vi "dB.vi"(8 "error in (no error)":errorcluster, 11 "Modulo a obtener":T1=enum."Error") -> (0 "error out":errorcluster)   [LabVIEW 2020]
uses:
  Comunes/Controles/Lista Modulos.ctl
  Comunes/Controles/FGV Opciones.ctl
  Comunes/Controles/Sql.ctl
  Comunes/Comunicacion/Mensajes.lvlib
types:
  T1 = typedef "Lista Modulos.ctl" = enum16{"Math", "Error", "Front", "Database", "Nuevos items"}
  T2 = typedef "FGV Opciones.ctl" = enum16{"Get", "Create", "Destroy"}
  T3 = enum32{"Invalid", "Standard", "Closed", "Hidden", "Minimized", "Maximized"}
  T4 = typedef "Sql.ctl" = enum16{"Get zapatos", "Insrt Zapatos", "Insrt Elementos", "Borrar Elementos"}
  T5 = cluster{"Fecha de termino":timestamp, "Fecha de inicio":timestamp, "Modelo":string, "Talla":string, "Color":string}
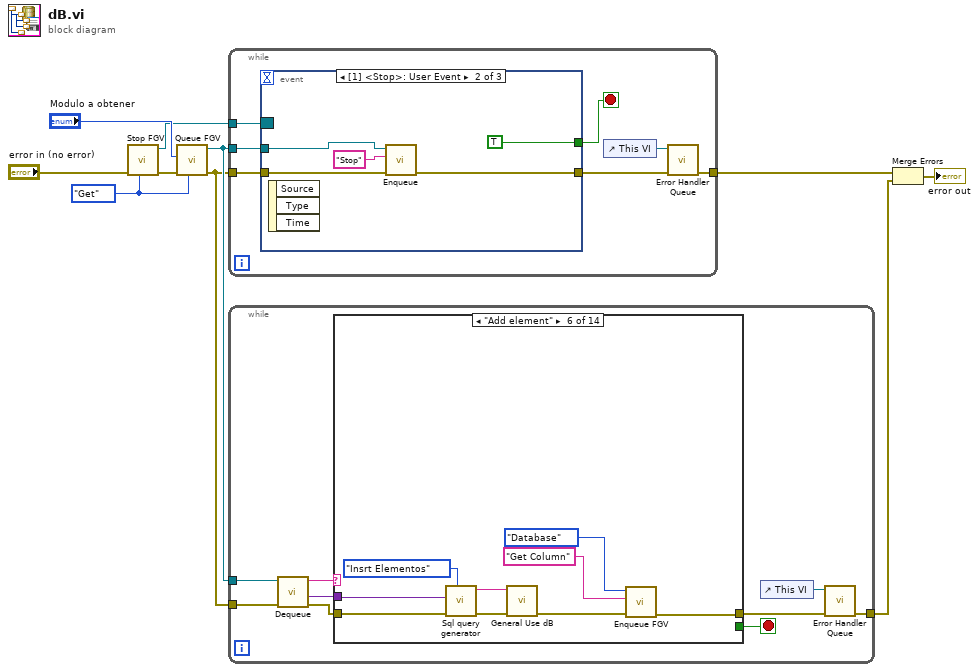
[diagram p0: block diagram]
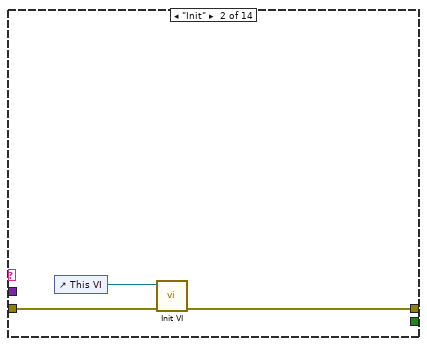
[diagram p3: hidden frame]
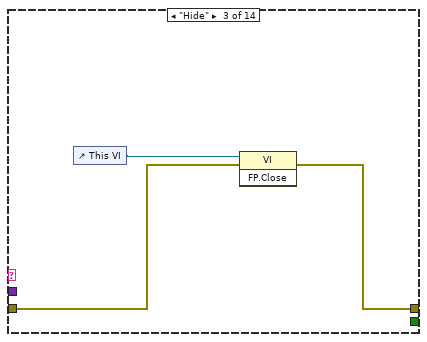
[diagram p4: hidden frame]
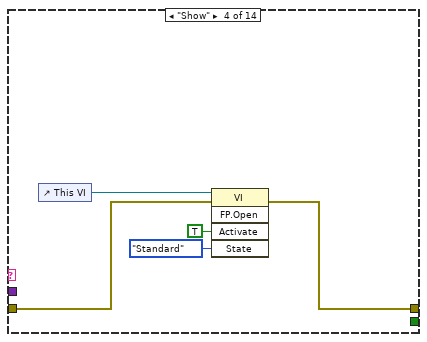
[diagram p5: hidden frame]
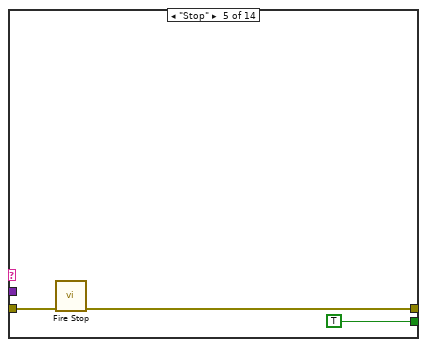
[diagram p6: hidden frame]
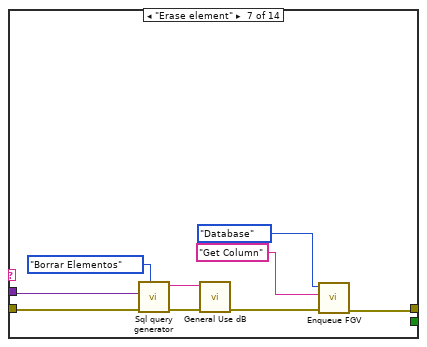
[diagram p7: hidden frame]
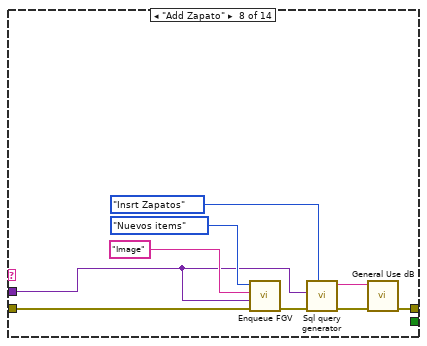
[diagram p8: hidden frame]
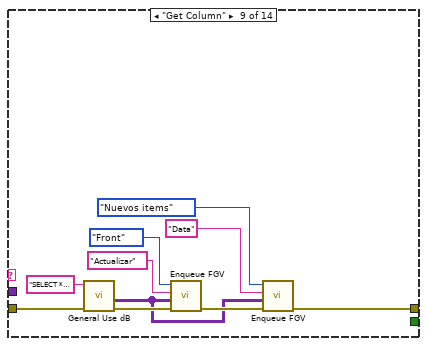
[diagram p9: hidden frame]
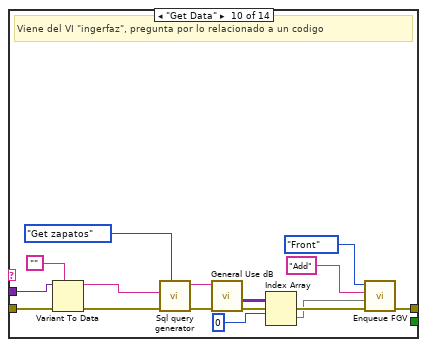
[diagram p10: hidden frame]
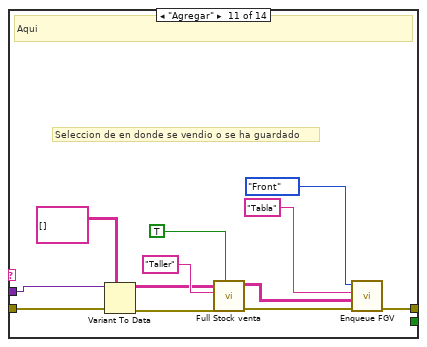
[diagram p11: hidden frame]
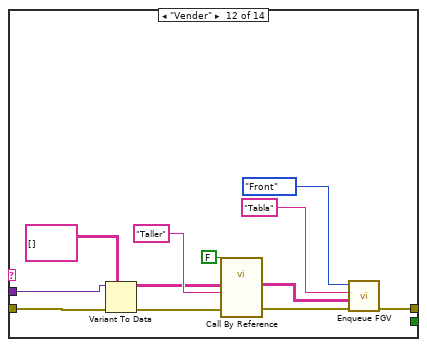
[diagram p12: hidden frame]
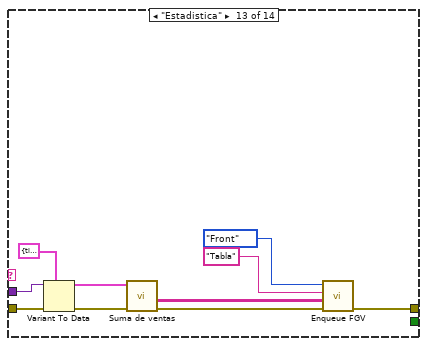
[diagram p13: hidden frame]
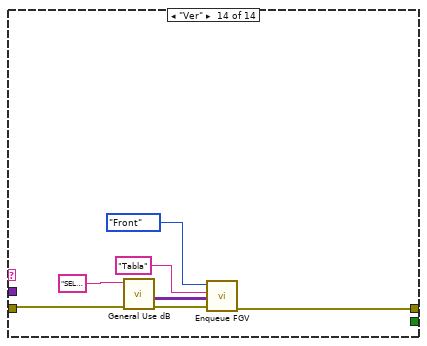
[diagram p14: hidden frame]
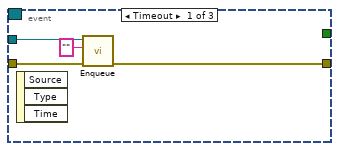
[diagram p15: hidden frame]
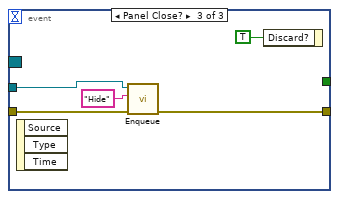
[diagram p16: hidden frame]
diagram:
  w1 = FGV_Opciones."Get" ("Enum")
  n1 = call "Stop FGV.vi"("Enum"=w1, "error in (no error)"="error in (no error)") -> ("error out"=w2:errorcluster, "Event Registration Refnum"=w4:refnum<event-registration>)  [unwired: 7 in, 1 out]
  n2 = call "Queue FGV.vi"("Enum"=w1, "error in (no error)"=w2, "Modulo a obtener"="Modulo a obtener") -> ("error out"=w8:errorcluster, "Queue Ref"=w9:refnum<queue>)  [unwired: 7 in]
  n3 = while {
    tunnel: w9 -> [w17]
    tunnel: w8 -> [w16]
    tunnel: [w14] -> w7
    tunnel: w4 -> [w12]
    stop <- w11 stop-if-true
    n4 = event shown="[1] <Stop>: User Event" {
      selector: w12 -> [_ _ _]
      dyn-events: _ -> [_ _ _]
      timeout: _ -> [_ _ _]
      tunnel: w17 -> [w21 w24 w30]
      tunnel: w16 -> [w20 w25 w29]
      tunnel: [w19 w22 w27] -> w13
      tunnel: [_ TRUE _] -> w11
      event Timeout {
        n5 = event-data() -> ()  [unwired: 1 in, 3 out]
        n6 = call "Enqueue.vi"("error in (no error)"=w20, "Mensaje"="", "Queue in"=w21) -> ("error out"=w19:errorcluster)  [unwired: 8 in]
      }
      event User Event {
        n7 = event-data() -> ()  [unwired: 1 in, 3 out]
        n8 = call "Enqueue.vi"("error in (no error)"=w25, "Mensaje"="Stop", "Queue in"=w24) -> ("error out"=w22:errorcluster)  [unwired: 8 in]
      }
      event Panel Close? {
        n9 = event-data() -> ()  [unwired: 1 in, 3 out]
        n10 = call "Enqueue.vi"("error in (no error)"=w29, "Mensaje"="Hide", "Queue in"=w30) -> ("error out"=w27:errorcluster)  [unwired: 8 in]
        n11 = event-data("Discard?"=TRUE) -> ()  [unwired: 1 in, 1 out]
      }
    }
    n12 = control-ref of="This VI"() -> (w15:refnum<vi>)
    n13 = call "Error Handler Queue.vi"("error in (no error)"=w13, "VI Refnum"=w15) -> ("error out"=w14:errorcluster)  [unwired: 9 in]
  }
  n14 = while {
    tunnel: w9 -> [w40]
    tunnel: w8 -> [w39]
    tunnel: [w33] -> w6
    stop <- w32 stop-if-true
    n15 = call "Dequeue.vi"("error in (no error)"=w39, "Queue in"=w40) -> ("error out"=w35:errorcluster, "Dato"=w37:variant, "Mensaje"=w38:string)  [unwired: 7 in]
    n16 = case shown="\"Add element\"" w38 {
      tunnel: w37 -> [_ _ _ _ _ w63 w66 w74 _ w106 w116 w127 w139 _]
      tunnel: w35 -> [w41 w44 w46 w49 w55 w64 w67 w78 w89 w107 w118 w129 w141 w148]
      tunnel: [w41 w43 w45 w48 w53 w58 w65 w79 w86 w98 w111 w121 w135 w142] -> w34
      tunnel: [_ _ _ _ TRUE _ _ _ _ _ _ _ _ _] -> w32
      frame "False", Default {
      }
      frame "Init" {
        n17 = control-ref of="This VI"() -> (w42:refnum<vi>)
        n18 = call "Init VI.vi"("error in (no error)"=w44, "VI in"=w42) -> ("error out"=w43:errorcluster)  [unwired: 9 in]
      }
      frame "Hide" {
        n19 = control-ref of="This VI"() -> (w47:refnum<vi>)
        n20 = invoke class="VI" method="FP.Close"(reference=w47, error in=w46) -> (error out=w45:errorcluster)  [unwired: 1 in, 2 out]
      }
      frame "Show" {
        n21 = control-ref of="This VI"() -> (w50:refnum<vi>)
        n22 = invoke class="VI" method="FP.Open"(reference=w50, error in=w49, "Activate"=TRUE ("Activate?"), "State"=T3."Standard") -> (error out=w48:errorcluster)  [unwired: 1 in, 4 out]
      }
      frame "Stop" {
        n23 = call "Fire Stop.vi"("error in (no error)"=w55) -> ("error out"=w53:errorcluster)  [unwired: 10 in]
      }
      frame "Add element" {
        n24 = call "Sql query generator.vi"("Modo"=Sql."Insrt Elementos", "error in"=w64, "Variant"=w63) -> ("error out"=w61:errorcluster, "Query"=w60:string)  [unwired: 7 in]
        n25 = call "General Use dB.vi"("error in (no error)"=w61, "Query"=w60) -> ("error out"=w59:errorcluster)  [unwired: 8 in, 1 out]
        n26 = call "Enqueue FGV.vi"("error in (no error)"=w59, "Mensaje"="Get Column", "Modulo a obtener"=Lista_Modulos."Database") -> ("error out"=w58:errorcluster)  [unwired: 8 in]
      }
      frame "Erase element" {
        n27 = call "Sql query generator.vi"("Modo"=Sql."Borrar Elementos", "error in"=w67, "Variant"=w66) -> ("error out"=w71:errorcluster, "Query"=w72:string)  [unwired: 7 in]
        n28 = call "General Use dB.vi"("error in (no error)"=w71, "Query"=w72) -> ("error out"=w73:errorcluster)  [unwired: 8 in, 1 out]
        n29 = call "Enqueue FGV.vi"("error in (no error)"=w73, "Mensaje"="Get Column", "Modulo a obtener"=Lista_Modulos."Database") -> ("error out"=w65:errorcluster)  [unwired: 8 in]
      }
      frame "Add Zapato" {
        n30 = call "Enqueue FGV.vi"("error in (no error)"=w78, "Dato"=w74, "Mensaje"="Image", "Modulo a obtener"=Lista_Modulos."Nuevos items") -> ("error out"=w77:errorcluster)  [unwired: 7 in]
        n31 = call "Sql query generator.vi"("Modo"=Sql."Insrt Zapatos", "error in"=w77, "Variant"=w74) -> ("error out"=w80:errorcluster, "Query"=w81:string)  [unwired: 7 in]
        n32 = call "General Use dB.vi"("error in (no error)"=w80, "Query"=w81) -> ("error out"=w79:errorcluster)  [unwired: 8 in, 1 out]
      }
      frame "Get Column" {
        n33 = call "General Use dB.vi"("error in (no error)"=w89, "Query"="SELECT * FROM Elementos") -> ("error out"=w90:errorcluster, "Return Data"=w83:variant[][])  [unwired: 8 in]
        n34 = call "Enqueue FGV.vi"("error in (no error)"=w90, "Dato"=w83, "Mensaje"="Actualizar", "Modulo a obtener"=Lista_Modulos."Front") -> ("error out"=w87:errorcluster)  [unwired: 7 in]
        n35 = call "Enqueue FGV.vi"("error in (no error)"=w87, "Dato"=w83, "Mensaje"="Data", "Modulo a obtener"=Lista_Modulos."Nuevos items") -> ("error out"=w86:errorcluster)  [unwired: 7 in]
      }
      frame "Get Data" {
        # "Viene del VI \"ingerfaz\", pregunta por lo relacionado a un codigo"
        n36 = Variant To Data(error in=w107, type="", Variant=w106) -> (data=w103:string, error out=w104:errorcluster)
        n37 = call "Sql query generator.vi"("Modo"=Sql."Get zapatos", "error in"=w104, "Variant"=w103) -> ("error out"=w101:errorcluster, "Query"=w100:string)  [unwired: 7 in]
        n38 = call "General Use dB.vi"("error in (no error)"=w101, "Query"=w100) -> ("error out"=w99:errorcluster, "Return Data"=w95:variant[][])  [unwired: 8 in]
        n39 = Index Array(array=w95, index (row)=0) -> (element=w93:variant[])  [unwired: 1 in]
        n40 = call "Enqueue FGV.vi"("error in (no error)"=w99, "Dato"=w93, "Mensaje"="Add", "Modulo a obtener"=Lista_Modulos."Front") -> ("error out"=w98:errorcluster)  [unwired: 7 in]
      }
      frame "Agregar" {
        # "Seleccion de en donde se vendio o se ha guardado"
        # "Aqui"
        n41 = Variant To Data(error in=w118, type=string[][] [] ("Value"), Variant=w116) -> (data=w114:string[][], error out=w117:errorcluster)
        n42 = call "Full Stock venta.vi"("Inventario/ventas"=TRUE, "error in (no error)"=w117, "Ubicacion"="Taller", "Full pedido"=w114) -> ("error out"=w112:errorcluster, "Sobrantes"=w110:string[][])  [unwired: 6 in]
        n43 = call "Enqueue FGV.vi"("error in (no error)"=w112, "Dato"=w110, "Mensaje"="Tabla", "Modulo a obtener"=Lista_Modulos."Front") -> ("error out"=w111:errorcluster)  [unwired: 7 in]
      }
      frame "Vender" {
        n44 = Variant To Data(error in=w129, type=string[][] [] ("Value"), Variant=w127) -> (data=w125:string[][], error out=w128:errorcluster)
        n45 = call-by-ref "?"("Inventario/ventas"=FALSE, "error in (no error)"=w128, "Ubicacion"="Taller", "Full pedido"=w125) -> ("error out"=w122:errorcluster, "Sobrantes"=w120:string[][])  [unwired: 8 in, 2 out]
        n46 = call "Enqueue FGV.vi"("error in (no error)"=w122, "Dato"=w120, "Mensaje"="Tabla", "Modulo a obtener"=Lista_Modulos."Front") -> ("error out"=w121:errorcluster)  [unwired: 7 in]
      }
      frame "Estadistica" {
        n47 = Variant To Data(error in=w141, type=T5 {"Fecha de termino"=timestamp(0 s since 1904-01-01), "Fecha de inicio"=timestamp(0 s since 1904-01-01), "Modelo"="", "Talla"="", "Color"=""} ("output cluster"), Variant=w139) -> (data=w137:T5, error out=w138:errorcluster)
        n48 = call "Suma de ventas.vi"("error in (no error)"=w138, "Input cluster"=w137) -> ("error out"=w136:errorcluster, "Array"=w134:string[][])  [unwired: 8 in]
        n49 = call "Enqueue FGV.vi"("error in (no error)"=w136, "Dato"=w134, "Mensaje"="Tabla", "Modulo a obtener"=Lista_Modulos."Front") -> ("error out"=w135:errorcluster)  [unwired: 7 in]
      }
      frame "Ver" {
        n50 = call "General Use dB.vi"("error in (no error)"=w148, "Query"="SELECT * FROM Inventario") -> ("error out"=w143:errorcluster, "Return Data"=w146:variant[][])  [unwired: 8 in]
        n51 = call "Enqueue FGV.vi"("error in (no error)"=w143, "Dato"=w146, "Mensaje"="Tabla", "Modulo a obtener"=Lista_Modulos."Front") -> ("error out"=w142:errorcluster)  [unwired: 7 in]
      }
    }
    n52 = control-ref of="This VI"() -> (w36:refnum<vi>)
    n53 = call "Error Handler Queue.vi"("error in (no error)"=w34, "VI Refnum"=w36) -> ("error out"=w33:errorcluster)  [unwired: 9 in]
  }
  n54 = Merge Errors(w7, w6) -> (→"error out":errorcluster)
